vi "Serialize Data.vi"(8 "error in (no error)":errorcluster, 11 "Process Data":T1) -> (0 "error out":errorcluster, 3 "Flat Data out":string)   [LabVIEW 2020, in "Unsigned Byte (U8).lvlib"]
doc: "Version 0.1"
uses:
  <vilib>/ADAS Record/CustomDataTypes/Unsigned Byte (U8)/Unsigned Byte (U8).lvlib
  <vilib>/ADAS Record/CustomDataTypes/Unsigned Byte (U8)/Process Data.ctl
  <vilib>/ADAS Record/IODataPEF/CfgMgr/FlatFormat.ctl
  69b4f655-d322-486f-8d65-ee31f7d8c6ef.vi
  <vilib>/ADAS Record/IODataPEF/Error/Error_CheckAndSetDllError.vi
  <vilib>/ADAS Record/IODataPEF/Error/Error_SetError.vi
  <vilib>/ADAS Record/IODataPEF/CfgMgr/GetPEFConfiguration_DefaultFlatFormat.vi
  <vilib>/ADAS Record/IODataPEF/Error/ErrorMgr.vi
  <vilib>/ADAS Record/CustomData/_Custom_RegisterType.vi
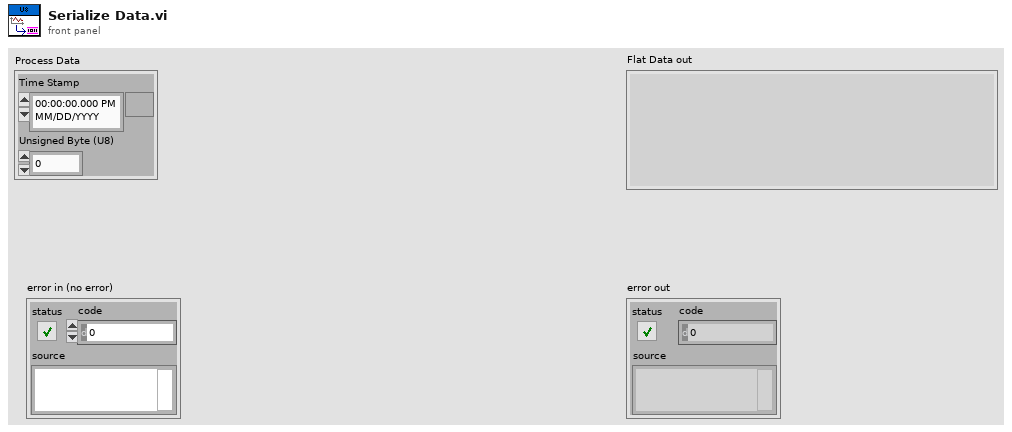
[diagram p1: front panel]
types:
  T1 = typedef "Unsigned Byte (U8).lvlib/Process Data.ctl" = cluster{"Time Stamp":timestamp, "Unsigned Byte (U8)":u8}
  T2 = typedef "FlatFormat.ctl" = enum32{"Auto", "PEF", "GFB (Apache)", "GFB", "JSON", "Readable JSON", "LV String", "Reserved", "LV Native"}
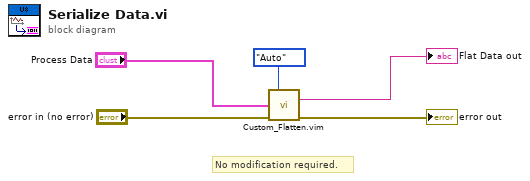
[diagram p0: block diagram]
diagram:
  # "No modification required."
  n1 = call "Custom_Flatten.vim"("Flat Format"=FlatFormat."Auto", "Data"="Process Data", "error in (no error)"="error in (no error)") -> ("Flat Data"=→"Flat Data out":string, "Error (out)"=→"error out":errorcluster)  [unwired: 10 in, 1 out]
